vi "WSL.vi"(0 "System no.":i32=1 min=1 max=4 step=1, 2 "Generator ID":i32[](array[numeric]) min=1 step=1, 3 "WaveTableID":i32[](array[numeric]), 5 "error in":errorcluster) -> (19 "error out":errorcluster)   [LabVIEW 2020]
doc: "Connects a wave table to a generator or disconnects the selected generator from any wave table.\n\nC-413: Generator ID can be 1 to 2, WaveTableID can be 1 to 8.\n\nC-886: Generator ID can be 1 to No. of connected axes, WaveTableID can be 1 to 100.\n\nC-887: Generator ID can be 1 to No. of connected axes, WaveTableID can be 1 to 100. \n\nC-891: Generator ID can be 1, WaveTableID can be 1 to 2.\n\nE-709: Generator ID can be 1, WaveTableID can be 1 to 6.\n\nE-517: Generator ID can be 1 to 3. WaveTableID can be 1 to 3. \n\nE-518: Generator ID can be 1 to 3. WaveTableID can be 1 to 3. \n\nE-712: Generator ID can be 1 to No. of connected axes, WaveTableID can be 1 to 90\n\nE-725: Generator ID can be 1 to No. of connected axes, WaveTableID can be 1 to 30\n\nE-727: Generator ID can be 1 to No. of connected axes, WaveTableID can be 1 to 40\n\nE-753: Generator ID can be 1, WaveTableID can be 1 to 10\n\nE-754: Generator ID can be 1, WaveTableID can be 1 to 10"
panel:
  # "Connects a wave table to a generator or, if WaveTableID is zero, \ndisconnects the selected generator from any wave table."
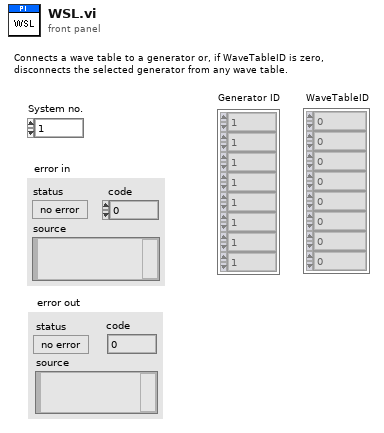
[diagram p1: front panel]
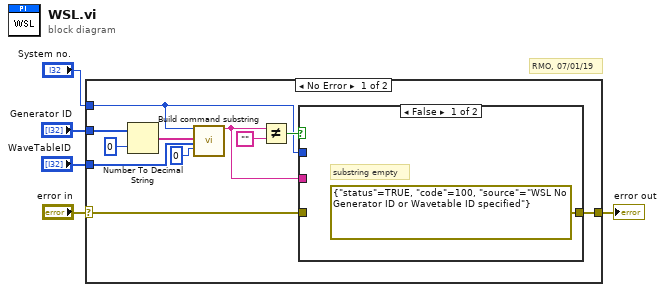
[diagram p0: block diagram]
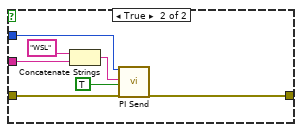
[diagram p2: hidden frame]
diagram:
  # "RMO, 07/01/19"
  n1 = case shown="No Error" "error in" {
    selector: "error in" -> [w6 w25]
    tunnel: [w16 w25] -> w5
    tunnel: "WaveTableID" -> [w13 _]
    tunnel: "System no." -> [w11 _]
    tunnel: "Generator ID" -> [w9 _]
    frame No Error {
      n2 = Number To Decimal String(number=w9, width (-)=i16 0) -> (decimal integer string=w10:string[])
      n3 = call "Build command substring.vi"("System no."=w11, "Affected axes"=w10, "Parameters"=w13, "No. of digits"=i16 0) -> ("Command substring"=w14:string)  [unwired: 3 in, 12 out]
      n4 = Not Equal?(x=w14, y="") -> (x != y?=w12:bool)
      n5 = case shown="False" w12 {
        tunnel: w14 -> [_ w23]
        tunnel: [errorcluster {"status"=TRUE, "code"=100, "source"="WSL No Generator ID or Wavetable ID specified"} ("error out") w18] -> w16
        tunnel: w6 -> [_ w20]
        tunnel: w11 -> [_ w19]
        frame False {
          # "substring empty"
        }
        frame True {
          n6 = Concatenate Strings("WSL", w23) -> (w21:string)
          n7 = call "PI Send.vi"("System no."=w19, "String to send"=w21, "Attach termination char.?"=TRUE ("Attach Linefeed?"), "error in"=w20) -> ("error out"=w18:errorcluster)  [unwired: 2 in, 13 out]
        }
      }
    }
    frame Error {
    }
  }
  "error out" <- w5
